vi "Normalize String.vi"(8 "error in":errorcluster, 9 "Normalized Form (C)":T1, 10 "Input Encoding (UTF-16LE)":T2=enum."UTF-16LE", 11 "String":string) -> (0 "error out":errorcluster, 3 "Normalized String":string)   [LabVIEW 2020, in "G-Unicode.lvlib"]
doc: "Normalizes <b>String</b> using the specified <b>Normalized Form</b>. Use this VI to normalize different representations of the same Unicode string into a single representation.\n\n<b>Note:</b> This function operates on 'raw' encoded strings. To normalize a UTF-8 String type, use Normalize String (Unicode).vim in the G-Unicode>String palette.\n\nSee this link for an in depth article on Unicode normalization:\nhttps://learn.microsoft.com/en-us/windows/win32/intl/using-unicode-normalization-to-represent-strings"
uses:
  G-Unicode.lvlib
  Controls/String Encoding.ctl
  String/Controls/Normalized Form.ctl
  Private/Conversion/Text to UTF-8.vi
  Private/Conversion/Polymorphic VIs/Text to UTF-8 (LabVIEW String).vi
  Private/Conversion/Encoded UTF-8 String to Encoded UTF-16LE String.vi
  SubVIs/UTF-16 Byte Swap.vi
  Private/Conversion/UTF-8 to Text.vi
  Private/Conversion/Polymorphic VIs/UTF-8 to Text (LabVIEW String).vi
  Private/Conversion/Encoded UTF-16LE String to Encoded UTF-8 String.vi
  Prepend BOM.vi
  Private/Memory/Copy String.vi
  Private/Library/Result To Error.vi
  SubVIs/Byte Order Marks.vi
  Detect BOM.vi
  Private/Memory/Copy String.vi/4d47babd-4a2d-4eb7-b91b-7e707d692665.vi
  Private/Library/gu_free.vi
  <vilib>/Utility/error.llb/Error Cluster From Error Code.vi
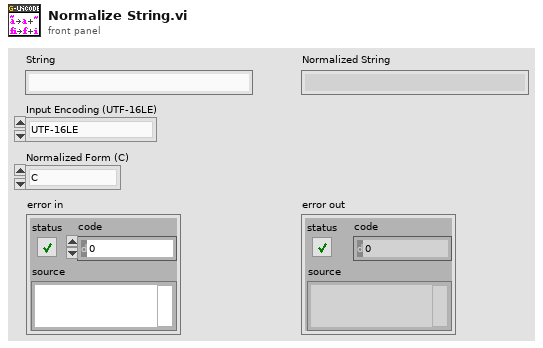
[diagram p1: front panel]
types:
  T1 = typedef "G-Unicode.lvlib/Normalized Form.ctl" = enum16{"C", "D", "KC", "KD"}
  T2 = typedef "G-Unicode.lvlib/String Encoding.ctl" = enum16{"ANSI", "UTF-8", "UTF-16LE", "UTF-16BE", "Unknown"}
  T3 = typedef "G-Unicode.lvlib/Encoded UTF-8 String.ctl" = string
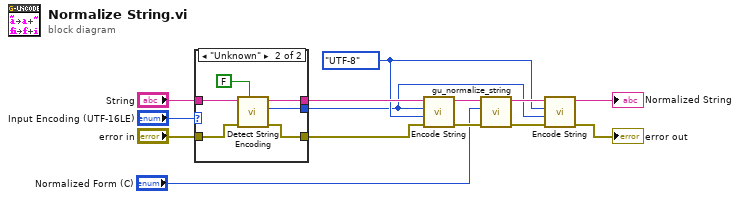
[diagram p0: block diagram]
diagram:
  w5 = String_Encoding."UTF-8" ("Output Encoding (UTF-16LE)")
  n1 = case shown="\"Unknown\"" "Input Encoding (UTF-16LE)" {
    selector: "Input Encoding (UTF-16LE)" -> [w15 _]
    tunnel: "String" -> [w17 w23]
    tunnel: [w15 w22] -> w4
    tunnel: [w17 w21] -> w11
    tunnel: "error in" -> [w16 w18]
    tunnel: [w16 w19] -> w10
    frame Default {
    }
    frame "Unknown" {
      n2 = call "Detect String Encoding.vi"("Strip BOM (T)"=FALSE ("Remove BOM (T)"), "error in"=w18, "String"=w23) -> ("error out"=w19:errorcluster, "Encoding"=w22:T2, "String out"=w21:string)  [unwired: 6 in]
    }
  }
  n3 = call "Encode String.vi"("error in"=w10, "Output Encoding (UTF-16LE)"=w5, "Input Encoding (ANSI)"=w4, "String in"=w11) -> ("error out"=w8:errorcluster, "String out"=w9:string)  [unwired: 6 in]
  n4 = call "gu_normalize_string.vi"("error in"=w8, "Normalized Form"="Normalized Form (C)", "String"=w9) -> ("error out"=w3:errorcluster, "Normalized String"=w6:T3)  [unwired: 7 in]
  n5 = call "Encode String.vi"("error in"=w3, "Output Encoding (UTF-16LE)"=w4, "Input Encoding (ANSI)"=w5, "String in"=w6) -> ("error out"=→"error out":errorcluster, "String out"=→"Normalized String":string)  [unwired: 6 in]
